vi "Set FIFO Flags.vi"(10 "FIFO":refnum<class "Debug Flags FIFO.lvclass">, 11 "Debug Flags in":refnum<class "Debug Flags.lvclass">) -> (3 "Debug Flags out":refnum<class "Debug Flags.lvclass">)   [LabVIEW 2017, in "Data Sharing Framework Engine.lvlib" / "Debug Flags.lvclass"]
uses:
  Debug Flags.lvclass
  Debug Flags FIFO/Debug Flags FIFO.lvclass
  Debug Flags.lvclass/Debug Flags.ctl
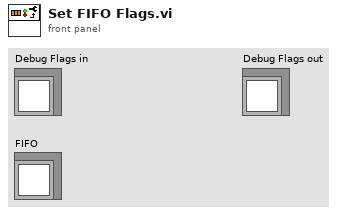
[diagram p1: front panel]
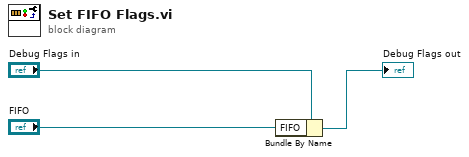
[diagram p0: block diagram]
diagram:
  n1 = Bundle By Name(cluster="Debug Flags in", "FIFO"="FIFO") -> (→"Debug Flags out":refnum<class "Debug Flags.lvclass">)
